vi "checkLowerBound.vi"(8 "yClick":i16, 9 "xClick":i16, 10 "yDimension":i16, 11 "xDimension":i16) -> (2 "yStart":i16, 3 "xStart":i16)   [LabVIEW 2016]
doc: "Check the ROI position is valid."
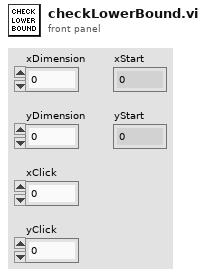
[diagram p1: front panel]
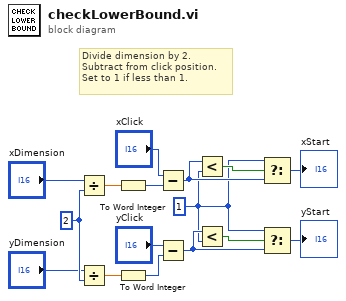
[diagram p0: block diagram]
diagram:
  w8 = i16 2
  w1 = i16 1 ("t")
  # "Divide dimension by 2.\nSubtract from click position.\nSet to 1 if less than 1."
  n1 = Divide(x="xDimension", y=w8) -> (x/y=w7:dbl)
  n2 = Divide(x="yDimension", y=w8) -> (x/y=w6:dbl)
  n3 = To Word Integer(number=w7) -> (16bit integer=w3:i16)
  n4 = To Word Integer(number=w6) -> (16bit integer=w2:i16)
  n5 = Subtract(x="xClick", y=w3) -> (x-y=w14:i16)
  n6 = Subtract(x="yClick", y=w2) -> (x-y=w13:i16)
  n7 = Less?(x=w14, y=w1) -> (x < y?=w11:bool)
  n8 = Less?(x=w13, y=w1) -> (x < y?=w12:bool)
  n9 = Select(t=w1, s=w11, f=w14) -> (s? t:f=→"xStart":i16)
  n10 = Select(t=w1, s=w12, f=w13) -> (s? t:f=→"yStart":i16)
